vi "saveSub.vi"(5 "Kanalnamen":string[](array[string]), 7 "Gruppenname":string, 8 "error":errorcluster, 10 "new data":dbl[][](array[numeric]), 11 "tdms file":refnum<k34>) -> (0 "error out":errorcluster, 3 "tdms file out":refnum<k34>)   [LabVIEW 2010, in "Licor-Steuerung.lvlib"]
uses:
  Licor-Steuerung.lvlib
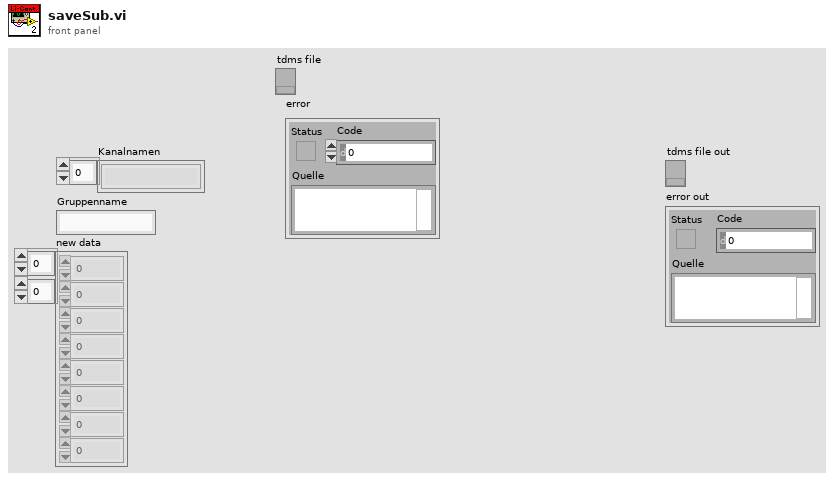
[diagram p1: front panel]
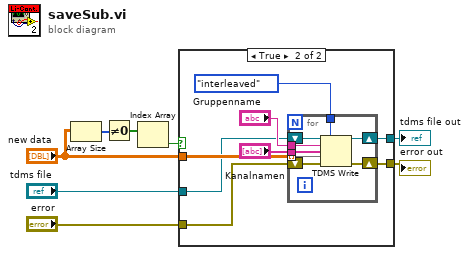
[diagram p0: block diagram]
diagram:
  n1 = Array Size(array="new data") -> (size(s)=w8:i32[])
  n2 = Not Equal To 0?(x=w8) -> (x != 0?=w2:bool[])
  n3 = Index Array(array=w2) -> (element=w1:bool)  [unwired: 1 in]
  n4 = case shown="True" w1 {
    tunnel: "new data" -> [_ w18]
    tunnel: "tdms file" -> [w10 w15]
    tunnel: "error" -> [w9 w14]
    tunnel: [w10 w12] -> w7
    tunnel: [w9 w11] -> w6
    frame False {
    }
    frame True {
      n5 = for {
        tunnel: w18 -> [w26] mode=indexing
        tunnel: "Kanalnamen" -> [w25]
        tunnel: "Gruppenname" -> [w24]
        tunnel: enum16{"decimated", "interleaved"}."interleaved" ("Daten-Layout (0:dezimiert)") -> [w21]
        shift-right: [w20] -> w12
        shift-left: w15 -> [w23]
        shift-right: [w19] -> w11
        shift-left: w14 -> [w22]
        n6 = TDMS Write(0:w23, 1:w21, 5:w24, 7:w25, 9:w26, 11:w22) -> (4:w20:refnum<k34>, 15:w19:errorcluster)  [unwired: 2 out]
      }
    }
  }
  "tdms file out" <- w7
  "error out" <- w6
